vi "disorder study.vi"() -> ()   [LabVIEW 2023]
uses:
  dllparameter.ctl
panel:
  in  "Disorder avg level":dbl=1.0
  out "Disorder":cluster{"Array":dbl[], "disorder":dbl[]}(graph)={"Array"=[0.0, 0.005, 0.01, 0.015, 0.02, 0.025, 0.03, 0.035, 0.04, 0.045, 0.05, 0.055, 0.06, 0.065, 0.07, 0.075, 0.08, 0.085, 0.09, 0.095, 0.1, 0.105, 0.11, 0.115, 0.12, 0.125, 0.13, 0.135, 0.14, 0.145, 0.15, 0.155, 0.16, 0.165, 0.17, 0.17500000000000002, 0.18, 0.185, 0.19, 0.195, 0.2, 0.20500000000000002, 0.21, 0.215, 0.22, 0.225, 0.23, 0.23500000000000001, 0.24, 0.245, 0.25, 0.255, 0.26, 0.265, 0.27, 0.275, 0.28, 0.28500000000000003, 0.29, 0.295, 0.3, 0.305, 0.31, 0.315, 0.32, 0.325, 0.33, 0.335, 0.34, 0.34500000000000003, 0.35000000000000003, 0.355, 0.36, 0.365, 0.37, 0.375, 0.38, 0.385, 0.39, 0.395, 0.4, 0.405, 0.41000000000000003, 0.41500000000000004, 0.42, 0.425, 0.43, 0.435, 0.44, 0.445, 0.45, 0.455, 0.46, 0.465, 0.47000000000000003, 0.47500000000000003, 0.48, 0.485, 0.49, 0.495, 0.5, 0.505, 0.51, 0.515, 0.52, 0.525, 0.53, 0.535, 0.54, 0.545, 0.55, 0.555, 0.56, 0.5650000000000001, 0.5700000000000001, 0.5750000000000001, 0.58, 0.585, 0.59, 0.595, 0.6, 0.605, 0.61, 0.615, 0.62, 0.625, 0.63, 0.635, 0.64, 0.645, 0.65, 0.655, 0.66, 0.665, 0.67, 0.675, 0.68, 0.685, 0.6900000000000001, 0.6950000000000001, 0.7000000000000001, 0.705, 0.71, 0.715, 0.72, 0.725, 0.73, 0.735, 0.74, 0.745, 0.75, 0.755, 0.76, 0.765, 0.77, 0.775, 0.78, 0.785, 0.79, 0.795, 0.8, 0.805, 0.81, 0.8150000000000001, 0.8200000000000001, 0.8250000000000001, 0.8300000000000001, 0.835, 0.84, 0.845, 0.85, 0.855, 0.86, 0.865, 0.87, 0.875, 0.88, 0.885, 0.89, 0.895, 0.9, 0.905, 0.91, 0.915, 0.92, 0.925, 0.93, 0.935, 0.9400000000000001, 0.9450000000000001, 0.9500000000000001, 0.9550000000000001, 0.96, 0.965, 0.97, 0.975, 0.98, 0.985, 0.99, 0.995, 1.0], "disorder"=[1.0, 1.0, 1.0, 1.0, 1.0, 1.0, 1.0, 1.0, 1.0, 1.0, 1.0, 1.0, 1.0, 1.0, 1.0, 1.0, 1.0, 1.0, 1.0, 1.0, 1.0, 1.1, 1.1, 1.1, 1.1, 1.1, 1.1, 1.1, 1.1, 1.1, 1.1, 1.1, 1.1, 1.1, 1.1, 1.1, 1.1, 1.1, 1.1, 1.1, 1.1, 1.0, 1.0, 1.0, 1.0, 1.0, 1.0, 1.0, 1.0, 1.0, 1.0, 1.0, 1.0, 1.0, 1.0, 1.0, 1.0, 1.0, 1.0, 1.0, 1.0, 1.0, 1.0, 1.0, 1.0, 1.0, 1.0, 1.0, 1.0, 1.0, 1.0, 1.0, 1.0, 1.0, 1.0, 1.0, 1.0, 1.0, 1.0, 1.0, 1.0, 1.0, 1.0, 1.0, 1.0, 1.0, 1.0, 1.0, 1.0, 1.0, 1.0, 1.0, 1.0, 1.0, 1.0, 1.0, 1.0, 1.0, 1.0, 1.0, 1.0, 1.0, 1.0, 1.0, 1.0, 1.0, 1.0, 1.0, 1.0, 1.0, 1.0, 1.0, 1.0, 1.0, 1.0, 1.0, 1.0, 1.0, 1.0, 1.0, 1.0, 1.0, 1.0, 1.0, 1.0, 1.0, 1.0, 1.0, 1.0, 1.0, 1.0, 1.0, 1.0, 1.0, 1.0, 1.0, 1.0, 1.0, 1.0, 1.0, 1.0, 1.0, 1.0, 1.0, 1.0, 1.0, 1.0, 1.0, 1.0, 1.0, 1.0, 1.0, 1.0, 1.0, 1.0, 1.0, 1.0, 1.0, 1.0, 1.0, 1.0, 1.0, 1.0, 1.0, 1.0, 1.0, 1.0, 1.0, 1.0, 1.0, 1.0, 1.0, 1.0, 1.0, 1.0, 1.0, 1.0, 1.0, 1.0, 1.0, 1.0, 1.0, 1.0, 1.0, 1.0, 1.0, 1.0, 1.0, 1.0, 1.0, 1.0, 1.0, 1.0, 1.0, 1.0, 1.0, 1.0, 1.0, 1.0, 1.0, 1.0]}
  in  "Disorder setting":enum32{"Flat disorder", "Bump", "3 ramps"}(tab)=enum."Bump"
  in  "bump amp":dbl=0.1
  in  "length percent":dbl=0.1
  in  "begin percent":dbl=0.1
  in  "P1 x":dbl=0.2
  in  "P1 y":dbl=0.1
  in  "P2 x":dbl=0.8
  in  "P2 y":dbl=0.1
  out "phaserange in Pi":i32=2
  out "pn0":dbl=-0.5
  out "pp0":dbl=0.5
  out "Diffraction pattern":cluster{dbl[], dbl[]}[](graph)
  out "Remaining steps":i32
  in  "flux step":dbl=0.01
  in  "flux end":dbl=10.0
  in  "flux start":dbl
  in  "Phase steps":i32=1001
  in  "Geometry steps":i32=1001
  # "Notes: use this VI to simulate diffraction of different geometry disorders."
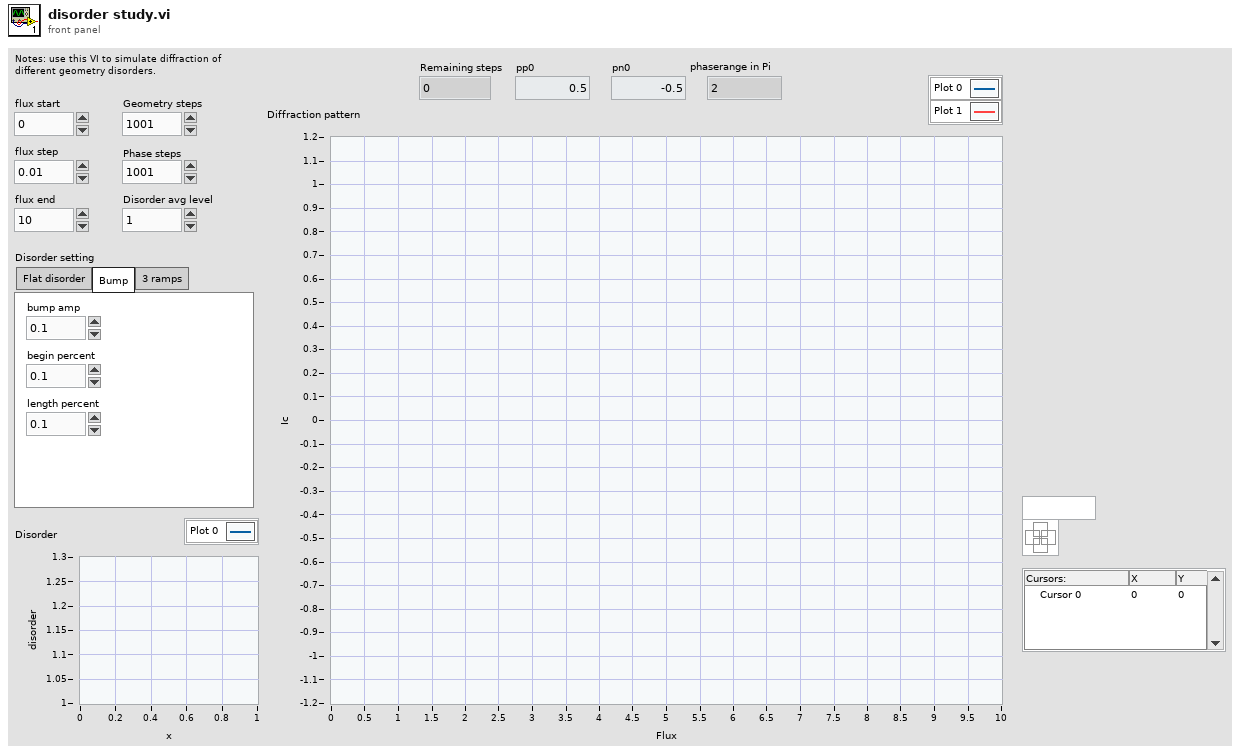
[diagram p1: front panel]
types:
  T1 = enum16{"Regular Josephson effect", "Non-local MBS", "Local MBS same parity", "Local MBS different parity"}
  T2 = typedef "dllparameter.ctl" = cluster{"Gaussian width":dbl, "Strenth of MBS":dbl, "Phase steps":i32, "Geometry steps":i32, "Geometry Noise Type":u16, "CPR Type":dbl, "parity for positive phase":dbl[], "parity for negative phase ":dbl[]}
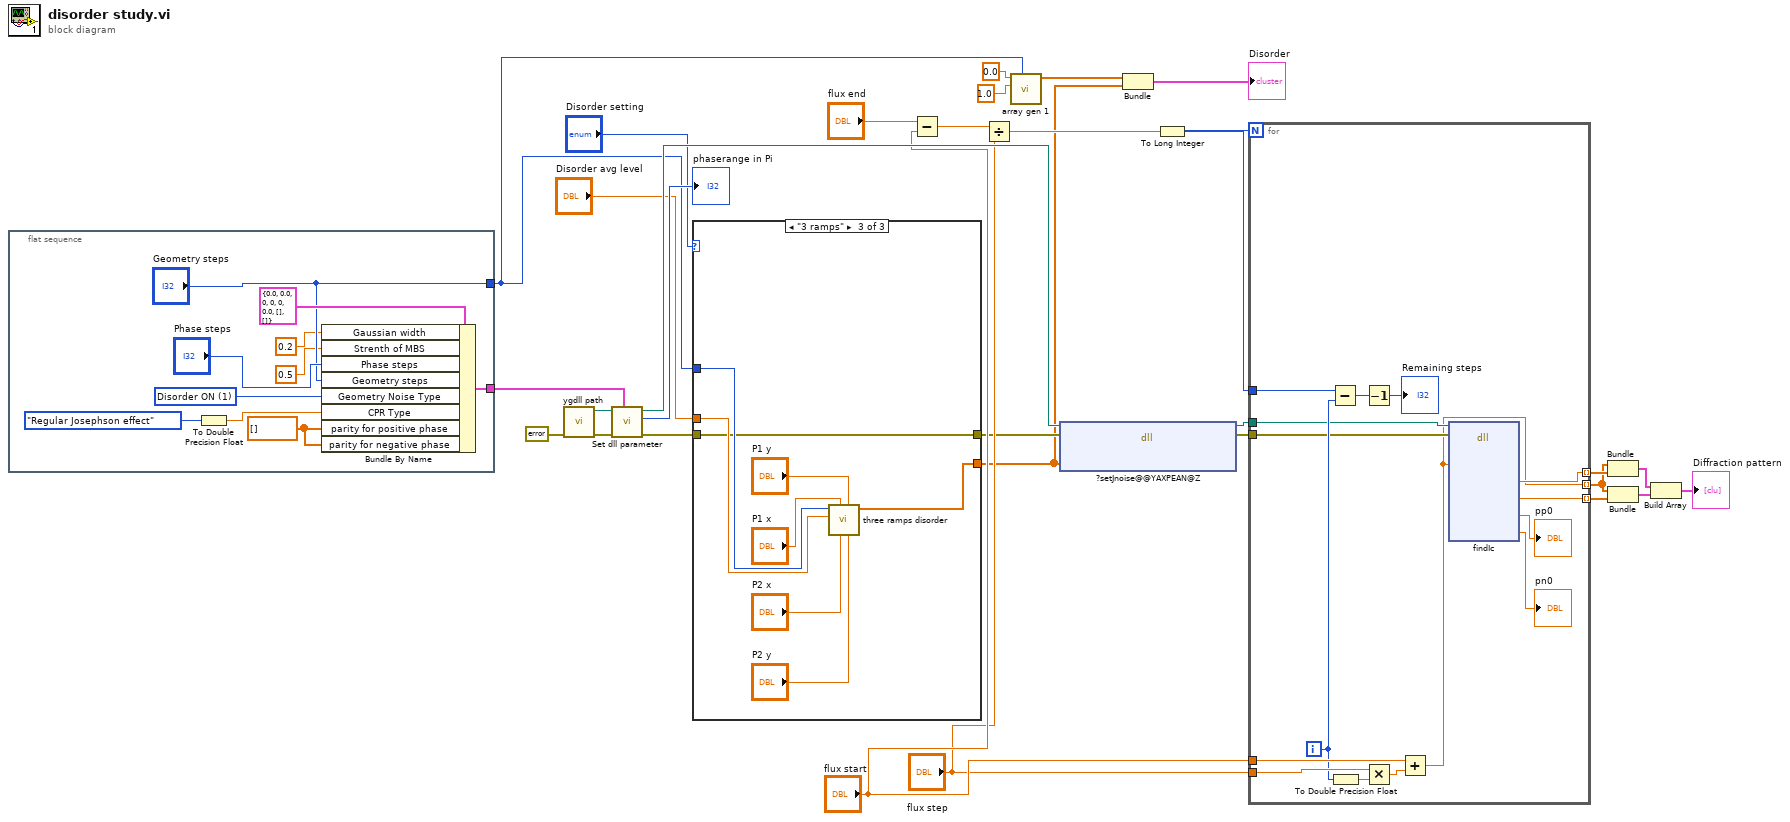
[diagram p0: block diagram]
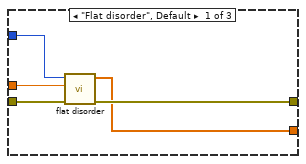
[diagram p2: hidden frame]
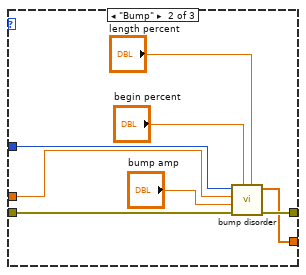
[diagram p3: hidden frame]
diagram:
  n1 = flat-sequence {
    tunnel: [w34] -> w27
    tunnel: ["Geometry steps"] -> w5
    frame #0 {
      w39 = u16 1 items=["Disorder OFF", "Disorder ON"] ("Geometry Disorder Type")
      w36 = dbl[] [] ("parity for positive phase")
      n2 = To Double Precision Float(number=T1."Regular Josephson effect" ("CPR Type")) -> (double precision float=w35:dbl)
      n3 = Bundle By Name(cluster=T2 {"Gaussian width"=0.0, "Strenth of MBS"=0.0, "Phase steps"=0, "Geometry steps"=0, "Geometry Noise Type"=0, "CPR Type"=0.0, "parity for positive phase"=[], "parity for negative phase "=[]} ("output cluster"), "Gaussian width"=0.2, "Strenth of MBS"=0.5, "Phase steps"="Phase steps", "Geometry steps"="Geometry steps", "Geometry Noise Type"=w39, "CPR Type"=w35, "parity for positive phase"=w36, "parity for negative phase"=w36) -> (w34:T2)
    }
  }
  n4 = call "ygdll path.vi"("error in (no error)"=errorcluster {"status"=FALSE, "code"=0, "source"=""}) -> ("error out"=w29:errorcluster, "appended path"=w28:path)  [unwired: 9 in]
  n5 = call "Set dll parameter.vi"("Parameter Cluster"=w27, "error in (no error)"=w29, "path in"=w28) -> ("error out"=w9:errorcluster, "phaserange in Pi"=→"phaserange in Pi":i32, "path out"=w26:path)  [unwired: 6 in]
  n6 = case shown="\"3 ramps\"" "Disorder setting" {
    tunnel: w9 -> [w45 w50 w54]
    tunnel: w5 -> [w44 w52 w61]
    tunnel: [w43 w49 w54] -> w8
    tunnel: [w42 w48 w55] -> w3
    tunnel: "Disorder avg level" -> [w41 w53 w60]
    frame "Flat disorder", Default {
      n7 = call "flat disorder.vi"("error in"=w45, "level"=w41, "Points"=w44) -> ("error out"=w43:errorcluster, "disorder"=w42:dbl[])  [unwired: 7 in]
    }
    frame "Bump" {
      n8 = call "bump disorder.vi"("length percent"="length percent", "begin percent"="begin percent", "error in"=w50, "amp"="bump amp", "level"=w53, "Points"=w52) -> ("error out"=w49:errorcluster, "disorder"=w48:dbl[])  [unwired: 4 in]
    }
    frame "3 ramps" {
      n9 = call "three ramps disorder.vi"("P2 y"="P2 y", "P1 y"="P1 y", "P2 x"="P2 x", "P1 x"="P1 x", "level"=w60, "points"=w61) -> ("Array"=w55:dbl[])  [unwired: 5 in]
    }
  }
  n10 = Subtract(x="flux end", y="flux start") -> (x-y=w23:dbl)
  n11 = Divide(x=w23, y="flux step") -> (x/y=w21:dbl)
  n12 = call "array gen 1.vi"("Points"=w5, "End"=1.0, "Start"=0.0) -> ("Array"=w4:dbl[])  [unwired: 8 in]
  n13 = dll-call lib="C:/Users/Guang Yue/Desktop/S-TI-S-simulation-C-code/x64/Release/ygDLL.dll" fn="?setJnoise@@YAXPEAN@Z"(path in=w26, error in=w8, "disorder"=w3) -> (path out=w19:path, error out=w18:errorcluster)  [unwired: 3 in]
  n14 = Bundle("Array"=w4, "Array"=w3) -> (→"Disorder":cluster{"Array":dbl[], "Array":dbl[]})  [unwired: 1 in]
  n15 = To Long Integer(number=w21) -> (32bit integer=w20:i32)
  n16 = for {
    N: w20 -> [_]
    tunnel: "flux start" -> [w76]
    tunnel: "flux step" -> [w75]
    tunnel: w20 -> [w73]
    tunnel: [w69] -> w17 mode=indexing
    tunnel: [w68] -> w15 mode=indexing
    tunnel: w19 -> [w67]
    tunnel: w18 -> [w66]
    tunnel: [w62] -> w16 mode=indexing
    i -> [w72]
    n17 = Subtract(x=w73, y=w72) -> (x-y=w71:i32)
    n18 = To Double Precision Float(number=w72) -> (double precision float=w74:dbl)
    n19 = Decrement(x=w71) -> (x-1=→"Remaining steps":i32)
    n20 = Multiply(x=w75, y=w74) -> (x*y=w65:dbl)
    n21 = Add(x=w76, y=w65) -> (x+y=w62:dbl)
    n22 = dll-call lib="C:/Users/yg/Box/Guang Yue uiuc research box folder/computation/S-TI-S jj simulation c/Release/ygDLL.dll" fn="findIc"(path in=w67, error in=w66, "flux"=w62) -> ("inp"=w69:dbl, "icn"=w68:dbl, "pp0"=→"pp0":dbl, "pn0"=→"pn0":dbl)  [unwired: 7 in, 2 out]
  }
  n23 = Bundle(w16, w17) -> (w14:cluster{dbl[], dbl[]})  [unwired: 1 in]
  n24 = Bundle(w16, w15) -> (w13:cluster{dbl[], dbl[]})  [unwired: 1 in]
  n25 = Build Array(w14, w13) -> (→"Diffraction pattern":cluster{dbl[], dbl[]}[])
